vi "Teleop.vi"(10 "Match Info":T1={"Autonomous Elapsed Seconds"=0.0, "TeleOp Elapsed Seconds"=0.0, "Disabled Elapsed Seconds"=0.0, "Visited Autonomous"=FALSE, "Visited TeleOp"=FALSE, "Visited Disabled"=FALSE, "Autonomous Settings"={"Autonomous Style"=enum."Independent", "VI Refnum"=refnum}}, 11 "Call Context":T2) -> ()   [LabVIEW 2013]
doc: "This VI is called for each TeleOp packet received from the DS where the robot is not disabled. It is often used to read from the joysticks and update I/O or to update setpoints for timed control loops. It should complete and return within 20 milliseconds or it may miss DS packets."
uses:
  <vilib>/Rock Robotics/WPI/DriverStation/WPI_DriverStationDerivedRobotMode.ctl
  <vilib>/Rock Robotics/WPI/DriverStation/WPI_DriverStationMatch Info.ctl
  Robot Global Data.vi
  <vilib>/Rock Robotics/WPI/RobotDrive/WPI_RobotDriveGetSetRefNum.vi
  <vilib>/Rock Robotics/WPI/Joystick/WPI_JoystickGetSetRefNum.vi
  <vilib>/Rock Robotics/WPI/RobotDrive/WPI_RobotDriveArcadeDrive_Standard(NoSaturation).vi
  <vilib>/Rock Robotics/WPI/CAN/Jaguar/SubVIs/WPI_CANJaguar_StatusSelect.ctl
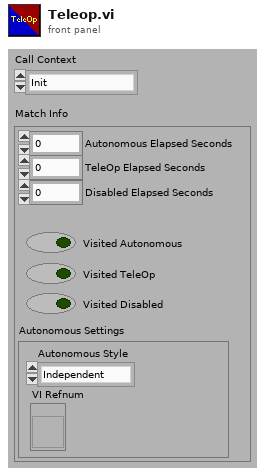
[diagram p1: front panel]
types:
  T1 = typedef "WPI_DriverStationMatch Info.ctl" = cluster{"Autonomous Elapsed Seconds":dbl, "TeleOp Elapsed Seconds":dbl, "Disabled Elapsed Seconds":dbl, "Visited Autonomous":bool, "Visited TeleOp":bool, "Visited Disabled":bool, "Autonomous Settings":cluster{"Autonomous Style":enum16{"Iterative", "Independent"}, "VI Refnum":refnum<vi>}}
  T2 = typedef "WPI_DriverStationDerivedRobotMode.ctl" = enum16{"Init", "Execute", "Stop"}
  T3 = typedef "WPI_RobotDriveDevRef.ctl" = cluster{"DevStatus":errorcluster, "Motors[]":T4[], "Square Inputs":bool, "Max Output":dbl, "Isochronous":bool}
  T4 = typedef "WPI_MotorControlDeviceRef.ctl" = cluster{"DeviceStatus":errorcluster, "Type":enum16{"PWM", "CAN"}, "PWM":cluster{"Digital Module":T5, "PWM Channel":T6, "DeadBand":T7}, "CAN":cluster{"Device Number":u8, "Control Mode":T8, "Semaphore":T9, "Max Vout":dbl}, "Invert":bool, "TransformRef":T10, "InvTransformRef":T10}
  T5 = typedef "FPGA_TypedefDigitalModule.ctl" = enum16{"Digital Module 1", "Digital Module 2"}
  T6 = typedef "FPGA_DIOPWMChannel.ctl" = enum8{"PWM 1", "PWM 2", "PWM 3", "PWM 4", "PWM 5", "PWM 6", "PWM 7", "PWM 8", "PWM 9", "PWM 10", "Invalid"}
  T7 = typedef "WPI_PWMDeadband.ctl" = cluster{"Name":string, "maxPositivePwm":i32, "minPositivePwm":i32, "centerPwm":i32, "maxNegativePwm":i32, "minNegativePwm":i32, "angularRange":u16}
  T8 = typedef "WPI_CANJaguar_ControlMode.ctl" = enum8{"Percent VBus", "Current", "Speed", "Position", "Voltage"}
  T9 = typedef "Semaphore RefNum" = refnum<k1>
  T10 = typedef "WPI_PWMTransform_ConPane.ctl" = refnum<vi>
  T11 = typedef "WPI_CANJaguar_StatusSelect.ctl" = enum16{"Output Percent VBus", "Output Voltage", "Bus Voltage", "Current", "Temperature", "Position", "Speed", "Limit Switches", "Faults", "Fault Counters", "Power Cycle"}
  T12 = typedef "WPI_CANJaguar_Status.ctl" = cluster{"Output Percent VBus":dbl, "Output Voltage":dbl, "Bus Voltage":dbl, "Current":dbl, "Temperature":dbl, "Position":dbl, "Speed":dbl, "Limits":cluster{"Forward Limit":bool, "Reverse Limit":bool, "Forward Soft Limit":bool, "Reverse Soft Limit":bool, "Sticky Forward Limit":bool, "Sticky Reverse Limit":bool, "Sticky Forward Soft Limit":bool, "Sticky Reverse Soft Limit":bool}, "Faults":cluster{"Current Fault":bool, "Temperature Fault":bool, "Bus Voltage Fault":bool, "Gate Driver Fault":bool, "Comm Fault":bool}, "Fault Counters":cluster{"Current Faults":u8, "Temperature Faults":u8, "Bus Voltage Faults":u8, "Gate Driver Faults":u8, "Comm Faults":u8, "CAN Status":u8, "CAN RX Errors":u8, "CAN TX Errors":u8}, "Power Cycle":bool}
  T13 = typedef "WPI_JoystickDevRef.ctl" = cluster{"Device":T14}
  T14 = typedef "WPI_JoystickDeviceEnum.ctl" = enum16{"USB 1", "USB 2", "USB 3", "USB 4", "Kinect 1", "Kinect 2"}
  T15 = cluster{"axis 1 (x)":dbl, "axis 2 (y)":dbl, "axis 3 (throttle)":dbl, "axis 4":dbl, "axis 5":dbl, "axis 6":dbl}
  T16 = cluster{"Left Motor Positions":cluster{"Low Extreme - 0 Degrees":dbl, "High Extreme - 180 Degrees":dbl}, "Right Motor Positions":cluster{"Low Extreme - 0 Degrees":dbl, "High Extreme - 180 Degrees":dbl}}
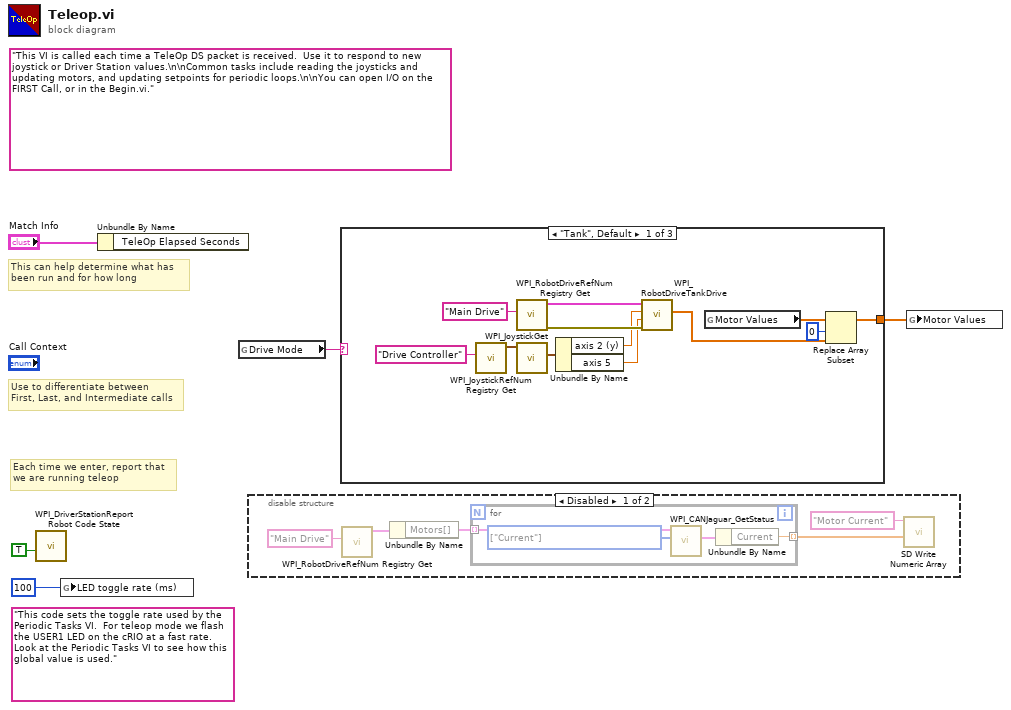
[diagram p0: block diagram]
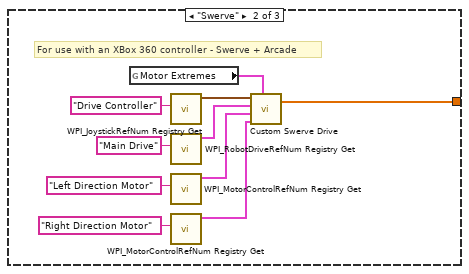
[diagram p3: hidden frame]
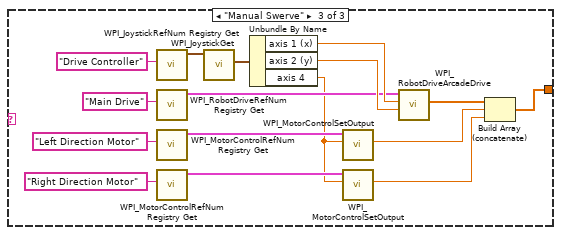
[diagram p4: hidden frame]
diagram:
  (unwired) "This code sets the toggle rate used by the Periodic Tasks VI.  For teleop mode we flash the USER1 LED on the cRIO at a fast rate.  Look at the Periodic Tasks VI to see how this global value is used."
  (unwired) "This VI is called each time a TeleOp DS packet is received.  Use it to respond to new joystick or Driver Station values.\n\nCommon tasks include reading the joysticks and updating motors, and updating setpoints for periodic loops.\n\nYou can open I/O on the FIRST Call, or in the Begin.vi."
  # "Each time we enter, report that\nwe are running teleop"
  # "Use to differentiate between\nFirst, Last, and Intermediate calls"
  # "This can help determine what has\nbeen run and for how long"
  n1 = call <vilib>:"WPI_DriverStationReport Robot Code State.vi"("TeleOp"=TRUE ("Autonomous")) -> ()  [unwired: 10 in, 1 out]
  n2 = global write "Robot Global Data.vi" "LED toggle rate (ms)"(u32 100 ("LED ms toggle rate")) -> ()
  n3 = Unbundle By Name("Match Info") -> ()  [unwired: 1 out]
  n4 = global read "Robot Global Data.vi" "Drive Mode"() -> (w2:string)
  n5 = disable-structure shown="Disabled" {
    frame Disabled {
      n6 = call <vilib>:"WPI_RobotDriveRefNum Registry Get.vi"("refnum name"="Main Drive") -> ("RobotDriveDevRef"=w9:T3)  [unwired: 9 in, 1 out]
      n7 = Unbundle By Name(w9) -> ("Motors[]"=w8:T4[])
      n8 = for {
        tunnel: w8 -> [w14] mode=indexing
        tunnel: [w11] -> w7 mode=indexing
        w13 = T11[] [enum."Current"] items=["Output Percent VBus", "Output Voltage", "Bus Voltage", "Current", "Temperature", "Position", "Speed", "Limit Switches", "Faults", "Fault Counters", "Power Cycle"] ("Status Select")
        n9 = call <vilib>:"WPI_CANJaguar_GetStatus.vi"("Status Select"=w13, "CAN Jaguar Ref"=w14) -> ("Status"=w12:T12)  [unwired: 7 in, 2 out]
        n10 = Unbundle By Name(w12) -> ("Current"=w11:dbl)
      }
      n11 = call <vilib>:"SD Write Numeric Array.vi"("Numeric Array"=w7, "Name"="Motor Current") -> ()  [unwired: 8 in, 2 out]
    }
    frame Enabled {
    }
  }
  n12 = case shown="\"Tank\", Default" w2 {
    tunnel: [w15 w27 w37] -> w1
    frame "Tank", Default {
      n13 = call <vilib>:"WPI_JoystickRefNum Registry Get.vi"("refnum name"="Drive Controller") -> ("JoystickDevRef"=w22:T13)  [unwired: 9 in, 1 out]
      n14 = call <vilib>:"WPI_RobotDriveRefNum Registry Get.vi"("refnum name"="Main Drive") -> ("error out"=w23:errorcluster, "RobotDriveDevRef"=w24:T3)  [unwired: 9 in]
      n15 = call <vilib>:"WPI_JoystickGet.vi"("JoystickDevRef"=w22) -> ("Axes"=w21:T15)  [unwired: 4 in, 2 out]
      n16 = Unbundle By Name(w21) -> ("axis 2 (y)"=w20:dbl, "axis 5"=w19:dbl)
      n17 = call <vilib>:"WPI_RobotDriveTankDrive.vi"("error in (no error)"=w23, "Right axis value"=w19, "Left axis value"=w20, "RobotDriveDevRef"=w24) -> ("Motor Values"=w16:dbl[])  [unwired: 5 in, 2 out]
      n18 = global read "Robot Global Data.vi" "Motor Values"() -> (w17:dbl[])
      n19 = Replace Array Subset(array=w17, new element=w16, index=0) -> (w15:dbl[])
    }
    frame "Swerve" {
      # "For use with an XBox 360 controller - Swerve + Arcade"
      n20 = global read "Robot Global Data.vi" "Motor Extremes"() -> (w30:T16)
      n21 = call <vilib>:"WPI_JoystickRefNum Registry Get.vi"("refnum name"="Drive Controller") -> ("JoystickDevRef"=w32:T13)  [unwired: 9 in, 1 out]
      n22 = call <vilib>:"WPI_RobotDriveRefNum Registry Get.vi"("refnum name"="Main Drive") -> ("RobotDriveDevRef"=w31:T3)  [unwired: 9 in, 1 out]
      n23 = call <vilib>:"WPI_MotorControlRefNum Registry Get.vi"("refnum name"="Left Direction Motor") -> ("MotorControlDevRef"=w29:T4)  [unwired: 9 in, 1 out]
      n24 = call <vilib>:"WPI_MotorControlRefNum Registry Get.vi"("refnum name"="Right Direction Motor") -> ("MotorControlDevRef"=w28:T4)  [unwired: 9 in, 1 out]
      n25 = call "Custom Swerve Drive.vi"("Motor Extremes"=w30, "Right Direction Motor Refnum"=w28, "Left Direction Motor Refnum"=w29, "Robot Drive Refnum"=w31, "Xbox Refnum"=w32) -> ("Motor Values"=w27:dbl[])  [unwired: 2 in]
    }
    frame "Manual Swerve" {
      n26 = call <vilib>:"WPI_JoystickRefNum Registry Get.vi"("refnum name"="Drive Controller") -> ("JoystickDevRef"=w48:T13)  [unwired: 9 in, 1 out]
      n27 = call <vilib>:"WPI_RobotDriveRefNum Registry Get.vi"("refnum name"="Main Drive") -> ("RobotDriveDevRef"=w44:T3)  [unwired: 9 in, 1 out]
      n28 = call <vilib>:"WPI_MotorControlRefNum Registry Get.vi"("refnum name"="Left Direction Motor") -> ("MotorControlDevRef"=w43:T4)  [unwired: 9 in, 1 out]
      n29 = call <vilib>:"WPI_MotorControlRefNum Registry Get.vi"("refnum name"="Right Direction Motor") -> ("MotorControlDevRef"=w42:T4)  [unwired: 9 in, 1 out]
      n30 = call <vilib>:"WPI_JoystickGet.vi"("JoystickDevRef"=w48) -> ("Axes"=w47:T15)  [unwired: 4 in, 2 out]
      n31 = Unbundle By Name(w47) -> ("axis 1 (x)"=w46:dbl, "axis 2 (y)"=w45:dbl, "axis 4"=w41:dbl)
      n32 = call <vilib>:"WPI_MotorControlSetOutput.vi"("Output"=w41, "MotorControlDevRef"=w43) -> ("Motor Output"=w39:dbl)  [unwired: 7 in, 2 out]
      n33 = call <vilib>:"WPI_MotorControlSetOutput.vi"("Output"=w41, "MotorControlDevRef"=w42) -> ("Motor Output"=w38:dbl)  [unwired: 7 in, 2 out]
      n34 = call-poly <vilib>:"WPI_RobotDriveArcadeDrive.vi"("Y axis value"=w45, "X axis value"=w46, "RobotDriveDevRef"=w44) -> ("Motor Values"=w40:dbl[])  [unwired: 6 in, 2 out]
      n35 = Build Array (concatenate)(w40, w39, w38) -> (w37:dbl[])
    }
  }
  n36 = global write "Robot Global Data.vi" "Motor Values"(w1) -> ()
